vi "RS.vi"(2 "SET":bool, 3 "RESET":bool) -> (1 "SAÍDA":bool)   [LabVIEW 2018]
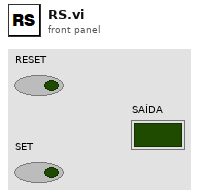
[diagram p1: front panel]
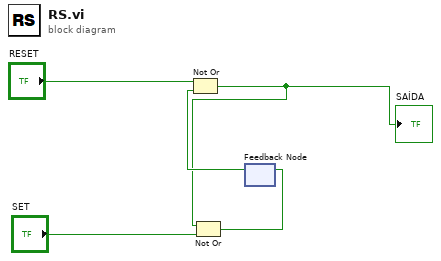
[diagram p0: block diagram]
diagram:
  n1 = feedback #1() -> (w2:bool)  [unwired: 1 in]
  n2 = Not Or(1:w2, 2:"RESET") -> (0:w1:bool)
  "SAÍDA" <- w1
  n3 = Not Or(1:"SET", 2:w1) -> (0:w3:bool)
  n4 = feedback-in #1(w3) -> ()
